vi "UnlinkNode.vi"(8 "error in":errorcluster, 10 "child in":T1, 11 "parent in":T1) -> (0 "error out":errorcluster, 2 "child out":T1, 3 "parent out":T1)   [LabVIEW 2013, in "NISE_CEF_Node.lvclass"]
doc: "Breaks the link between a child and a parent node. Removing the reference to each other in both nodes."
uses:
  NISE_CEF_Node.lvclass
  NodeRef.ctl
  NISE_CEF_Node.lvclass/NISE_CEF_Node.ctl
  ReadChildren.vi
  WriteParent.vi
  WriteChildren.vi
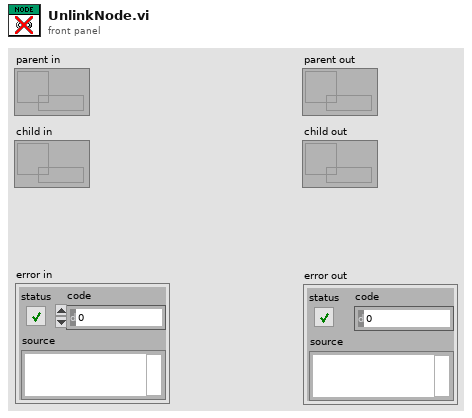
[diagram p1: front panel]
types:
  T1 = typedef "NISE_CEF_Node.lvclass/NodeRef.ctl" = refnum<data-value>
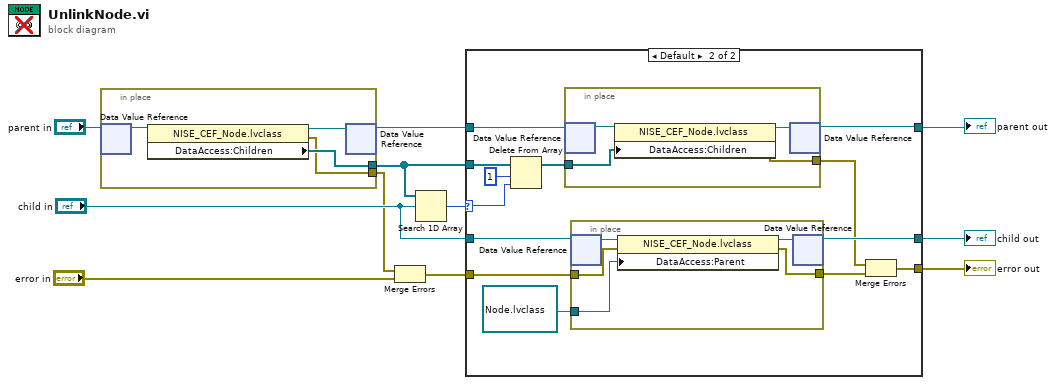
[diagram p0: block diagram]
diagram:
  n1 = in-place {
    in-place-border: [w13] -> w9
    in-place-border: [w12] -> w1
    n2 = in-place-dvr #1("parent in") -> (w15:refnum<class "NISE_CEF_Node.lvclass">)  [unwired: 1 out]
    n3 = property class="NISE_CEF_Node.lvclass"(reference=w15) -> (reference out=w14:refnum<class "NISE_CEF_Node.lvclass">, error out=w12:errorcluster, "DataAccess:Children"=w13:T1[])  [unwired: 1 in]
    n4 = in-place-dvr #1(w14) -> (w10:T1)  [unwired: 1 out]
  }
  n5 = Merge Errors(w1, "error in") -> (w2:errorcluster)
  n6 = Search 1D Array(1D array=w9, element="child in") -> (index of element=w11:i32)  [unwired: 1 in]
  n7 = case shown="Default" w11 {
    selector: w11 -> [_ w26]
    tunnel: "child in" -> [w16 w31]
    tunnel: w2 -> [w18 w30]
    tunnel: [w18 w20] -> w8
    tunnel: w10 -> [w17 w23]
    tunnel: [w17 w25] -> w4
    tunnel: [w16 w29] -> w5
    tunnel: w9 -> [_ w28]
    frame -1 {
    }
    frame Default {
      n8 = Delete From Array(array=w28, length=1, index=w26) -> (array with subset deleted=w24:T1[])  [unwired: 1 out]
      n9 = in-place {
        in-place-border: w24 -> [w33]
        in-place-border: [w32] -> w19
        n10 = in-place-dvr #2(w23) -> (w35:refnum<class "NISE_CEF_Node.lvclass">)  [unwired: 1 out]
        n11 = property class="NISE_CEF_Node.lvclass"(reference=w35, "DataAccess:Children"=w33) -> (reference out=w34:refnum<class "NISE_CEF_Node.lvclass">, error out=w32:errorcluster)  [unwired: 1 in]
        n12 = in-place-dvr #2(w34) -> (w25:T1)  [unwired: 1 out]
      }
      n13 = in-place {
        in-place-border: w30 -> [w39]
        in-place-border: refnum<data-value> refnum ("parent out") -> [w37]
        in-place-border: [w36] -> w21
        n14 = in-place-dvr #3(w31) -> (w40:refnum<class "NISE_CEF_Node.lvclass">)  [unwired: 1 out]
        n15 = property class="NISE_CEF_Node.lvclass"(reference=w40, error in=w39, "DataAccess:Parent"=w37) -> (reference out=w38:refnum<class "NISE_CEF_Node.lvclass">, error out=w36:errorcluster)
        n16 = in-place-dvr #3(w38) -> (w29:T1)  [unwired: 1 out]
      }
      n17 = Merge Errors(w19, w21) -> (w20:errorcluster)
    }
  }
  "child out" <- w5
  "parent out" <- w4
  "error out" <- w8
